vi "InteractiveStepperControl.vi"(8 "error in":errorcluster) -> ()   [LabVIEW 2015]
doc: "Commands\n 0 - set units (0-inHg, 1-mmHg, 2-torr, 3-mbar)\n 1 - set vacuum zero\n 2 - reserved\n 3 - reserved\n 4 - reserved\n 5 - set vacuum calibration\n 6 - reserved\n 7 - start bootloader\n 8 - get firmware version\n 9 - get vacuum reading\n 10 - start/stop vacuum control (0-stop, 1-start)\n 11 - set vacuum setpoint\n 12 - set calibration zero offset (prevent negative zero value from DWIN)\n 13 - set pump speed 0-100 \n 14 - set vacuum valve PWM 0-1000\n 15 - set bleed valve PWM 0-1000"
panel:
  in  "Move":bool
  in  "Hz":sgl=1.0 min=1 max=2000 step=1
  in  "Steps":sgl min=0 max=100000 step=1
  in  "Direction":bool
  in  "Enable":bool
  in  "stop":bool
  out "element":string
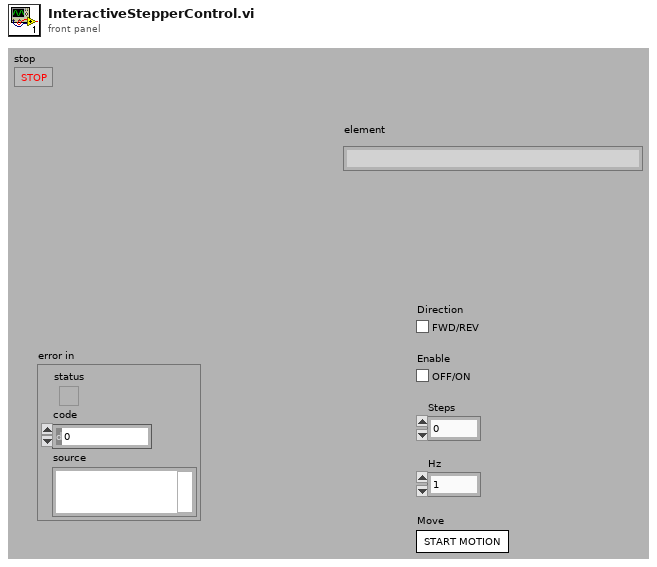
[diagram p1: front panel]
types:
  T1 = enum16{"usbSetEnable", "usbSetDirection", "usbSetCounts", "usbSetClock", "usbStartMotion"}
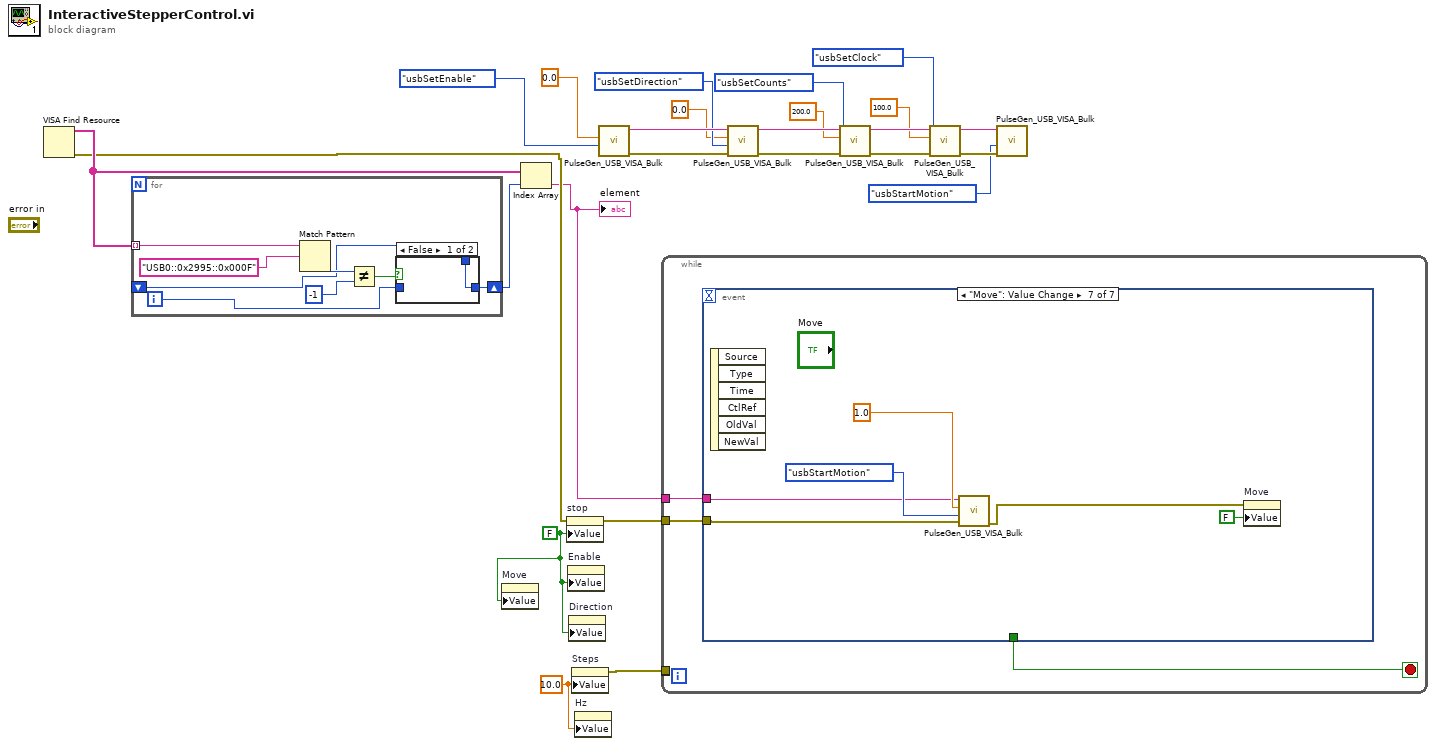
[diagram p0: block diagram]
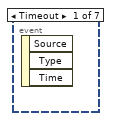
[diagram p2: hidden frame]
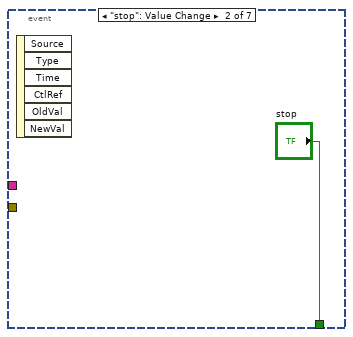
[diagram p3: hidden frame]
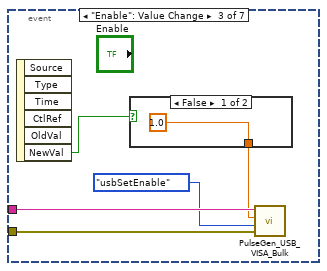
[diagram p4: hidden frame]
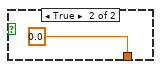
[diagram p5: hidden frame]
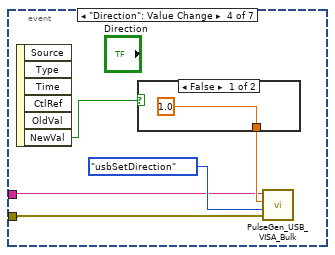
[diagram p6: hidden frame]
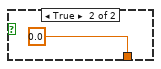
[diagram p7: hidden frame]
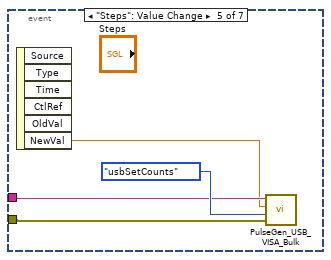
[diagram p8: hidden frame]
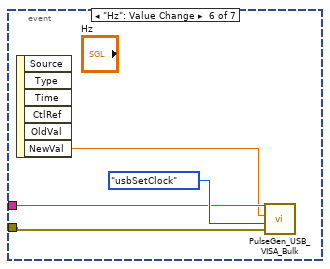
[diagram p9: hidden frame]
diagram:
  w2 = sgl 10.0 ("Steps")
  w1 = FALSE ("stop")
  n1 = VISA Find Resource() -> (0:w5:errorcluster, 3:w25:string[])  [unwired: 3 in, 1 out]
  n2 = for {
    tunnel: w25 -> [w33] mode=indexing
    shift-right: [w27] -> w24
    shift-left: _ -> [w26]
    i -> [w28]
    n3 = Match Pattern(string=w33, regular expression="USB0::0x2995::0x000F" ("element")) -> (offset past match=w31:i32)  [unwired: 1 in, 3 out]
    n4 = Not Equal?(x=w31, y=-1) -> (x != y?=w29:bool)
    n5 = case shown="False" w29 {
      tunnel: w28 -> [_ w35]
      tunnel: [w34 w35] -> w27
      tunnel: w26 -> [w34 _]
      frame False {
      }
      frame True {
      }
    }
  }
  n6 = property on="Move" class="Bool (strict)"("Value"=w1) -> ()  [unwired: 2 in, 2 out]
  n7 = Index Array(array=w25, index=w24) -> (element=w4:string)
  "element" <- w4
  n8 = property on="stop" class="Bool (strict)"(error in=w5, "Value"=w1) -> (error out=w6:errorcluster)  [unwired: 1 in, 1 out]
  n9 = property on="Enable" class="Bool (strict)"("Value"=w1) -> ()  [unwired: 2 in, 2 out]
  n10 = property on="Direction" class="Bool (strict)"("Value"=w1) -> ()  [unwired: 2 in, 2 out]
  n11 = property on="Steps" class="DigNum (strict)"("Value"=w2) -> (error out=w3:errorcluster)  [unwired: 2 in, 1 out]
  n12 = property on="Hz" class="DigNum (strict)"("Value"=w2) -> ()  [unwired: 2 in, 2 out]
  n13 = call "PulseGen_USB_VISA_Bulk.vi"("Command Index"=T1."usbSetEnable", "Numeric Input (Optional)"=sgl 0.0) -> ("error out"=w21:errorcluster, "Resource Name 2"=w20:string)  [unwired: 7 in, 1 out]
  n14 = while {
    tunnel: w6 -> [w38]
    tunnel: w4 -> [w37]
    tunnel: [w36] -> _
    tunnel: w3 -> [w36]
    stop <- w39 stop-if-true
    n15 = event shown="[6] \"Move\": Value Change" {
      selector: _ -> [_ _ _ _ _ _ _]
      dyn-events: _ -> [_ _ _ _ _ _ _]
      timeout: _ -> [_ _ _ _ _ _ _]
      tunnel: [_ "stop" _ _ _ _ _] -> w39
      tunnel: w38 -> [_ _ w45 w49 w56 w60 w64]
      tunnel: w37 -> [_ _ w44 w50 w57 w61 w65]
      event Timeout {
        n16 = event-data() -> ()  [unwired: 1 in, 3 out]
      }
      event "stop": Value Change {
        n17 = event-data() -> ()  [unwired: 1 in, 6 out]
      }
      event "Enable": Value Change {
        n18 = event-data() -> ("NewVal"=w42:bool)  [unwired: 1 in, 5 out]
        n19 = case shown="False" w42 {
          tunnel: [sgl 1.0 sgl 0.0] -> w41
          frame False {
          }
          frame True {
          }
        }
        n20 = call "PulseGen_USB_VISA_Bulk.vi"("error in"=w45, "Command Index"=T1."usbSetEnable", "Numeric Input (Optional)"=w41, "Resource Name"=w44) -> ()  [unwired: 5 in, 3 out]
      }
      event "Direction": Value Change {
        n21 = event-data() -> ("NewVal"=w48:bool)  [unwired: 1 in, 5 out]
        n22 = case shown="False" w48 {
          tunnel: [sgl 1.0 sgl 0.0] -> w51
          frame False {
          }
          frame True {
          }
        }
        n23 = call "PulseGen_USB_VISA_Bulk.vi"("error in"=w49, "Command Index"=T1."usbSetDirection", "Numeric Input (Optional)"=w51, "Resource Name"=w50) -> ()  [unwired: 5 in, 3 out]
      }
      event "Steps": Value Change {
        n24 = event-data() -> ("NewVal"=w55:sgl)  [unwired: 1 in, 5 out]
        n25 = call "PulseGen_USB_VISA_Bulk.vi"("error in"=w56, "Command Index"=T1."usbSetCounts", "Numeric Input (Optional)"=w55, "Resource Name"=w57) -> ()  [unwired: 5 in, 3 out]
      }
      event "Hz": Value Change {
        n26 = event-data() -> ("NewVal"=w59:sgl)  [unwired: 1 in, 5 out]
        n27 = call "PulseGen_USB_VISA_Bulk.vi"("error in"=w60, "Command Index"=T1."usbSetClock", "Numeric Input (Optional)"=w59, "Resource Name"=w61) -> ()  [unwired: 5 in, 3 out]
      }
      event "Move": Value Change {
        n28 = event-data() -> ()  [unwired: 1 in, 6 out]
        n29 = call "PulseGen_USB_VISA_Bulk.vi"("error in"=w64, "Command Index"=T1."usbStartMotion", "Numeric Input (Optional)"=sgl 1.0, "Resource Name"=w65) -> ("error out"=w63:errorcluster)  [unwired: 5 in, 2 out]
        n30 = property on="Move" class="Bool (strict)"(error in=w63, "Value"=FALSE ("Move")) -> ()  [unwired: 1 in, 2 out]
      }
    }
  }
  n31 = call "PulseGen_USB_VISA_Bulk.vi"("error in"=w21, "Command Index"=T1."usbSetDirection", "Numeric Input (Optional)"=sgl 0.0, "Resource Name"=w20) -> ("error out"=w17:errorcluster, "Resource Name 2"=w16:string)  [unwired: 5 in, 1 out]
  n32 = call "PulseGen_USB_VISA_Bulk.vi"("error in"=w17, "Command Index"=T1."usbSetCounts", "Numeric Input (Optional)"=sgl 200.0, "Resource Name"=w16) -> ("error out"=w13:errorcluster, "Resource Name 2"=w12:string)  [unwired: 5 in, 1 out]
  n33 = call "PulseGen_USB_VISA_Bulk.vi"("error in"=w13, "Command Index"=T1."usbSetClock", "Numeric Input (Optional)"=sgl 100.0, "Resource Name"=w12) -> ("error out"=w9:errorcluster, "Resource Name 2"=w8:string)  [unwired: 5 in, 1 out]
  n34 = call "PulseGen_USB_VISA_Bulk.vi"("error in"=w9, "Command Index"=T1."usbStartMotion", "Resource Name"=w8) -> ()  [unwired: 6 in, 3 out]
